vi "Write DVR.vi"(8 "error in (no error)":errorcluster, 10 "DVR":refnum<data-value>, 11 "PAS UI in":refnum<class "PAS UI.lvclass">) -> (0 "error out":errorcluster, 3 "PAS UI out":refnum<class "PAS UI.lvclass">)   [LabVIEW 2012, in "PAS UI.lvclass"]
uses:
  PAS UI.lvclass
  Data/cPAS Data.lvclass
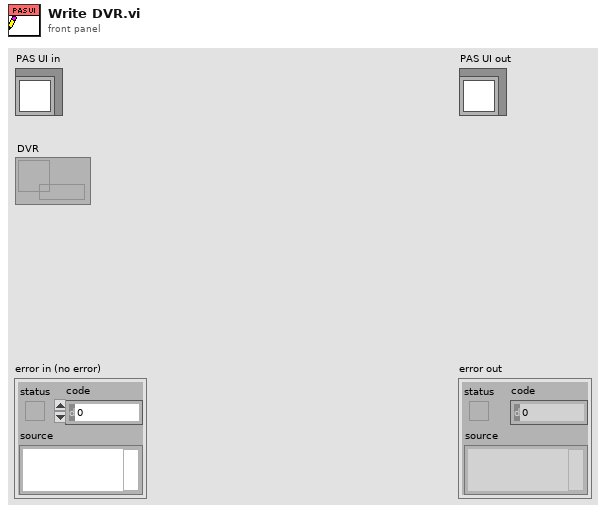
[diagram p1: front panel]
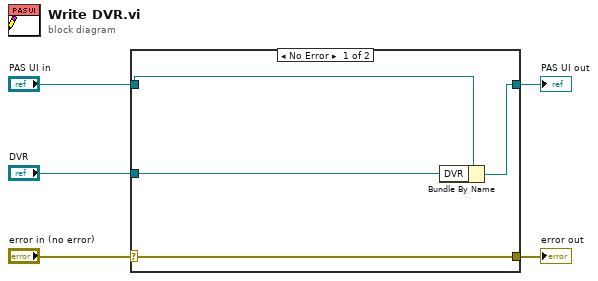
[diagram p0: block diagram]
diagram:
  n1 = case shown="No Error" "error in (no error)" {
    selector: "error in (no error)" -> [w9 w10]
    tunnel: [w9 w10] -> w4
    tunnel: [w7 w11] -> w2
    tunnel: "PAS UI in" -> [w8 w11]
    tunnel: "DVR" -> [w6 _]
    frame No Error {
      n2 = Bundle By Name(cluster=w8, "DVR"=w6) -> (w7:refnum<class "PAS UI.lvclass">)
    }
    frame Error {
    }
  }
  "error out" <- w4
  "PAS UI out" <- w2
